vi "Main.vi"() -> ()   [LabVIEW 2019, in "Server.lvlib"]
doc: "This template is based off of the Queued Message Handler design pattern and the Queued Message Handler project template that ships with LabVIEW.\n\nThe main difference is that the queue is private to this module and communication between modules is performed via Broadcast and Request events.\n\nRequest events are wrapped in public API methods and are handled in the Event Handling Loop (EHL) of this VI. Any module can register for Broadcast events sent by this module. The EHL generates messages based on user interface actions.\n\nThe Message Handling Loop (MHL) processes messages generated by the EHL, or by other messages. The messages are string values, so new messages can be added easily to the Message Cases case structure in the MHL. Each message cluster can also provide an optional value for Message Data, which is a variant that can be converted to whatever message-specific data is required.\n_____\nBased on Delacor QMH Project Template 4.2.1.64."
uses:
  Server.lvlib
  <vilib>/Delacor/Delacor QMH/Libraries/Module Admin_class/Delacor_lib_QMH_Module Admin.lvclass
  Module Data--cluster.ctl
  <vilib>/Delacor/Delacor QMH/Libraries/Message Queue_class/Delacor_lib_QMH_Message Queue.lvclass/Delacor_lib_QMH_Message Queue.ctl
  Stop Argument--cluster.ctl
  <vilib>/Delacor/Delacor QMH/Libraries/Module Admin_class/Delacor_lib_QMH_Module Admin.lvclass/Delacor_lib_QMH_Module Admin.ctl
  <vilib>/Utility/miscctls.llb/LVPointTypeDef.ctl
  <vilib>/Delacor/Delacor QMH/Libraries/Message Queue_class/Delacor_lib_QMH_Enqueue Message (Single).vi
  <vilib>/Delacor/Delacor QMH/Libraries/Module Admin_class/Delacor_lib_QMH_Get External Launch.vi
  <vilib>/Utility/error.llb/Error Cluster From Error Code.vi
  <vilib>/ErrorRing/Error Ring.xnode
  <vilib>/Delacor/Delacor QMH/Libraries/Message Queue_class/Delacor_lib_QMH_Message Queue.lvclass
  Chat Window/Chat Window.lvlib
panel:
  in  "Chat Window Selection":i32(ring) items=["All"=-1]
  in  "Send Global Chat":bool
  in  "New Chat Window":bool
  in  "Send Message":string
  in  "Simulate MHL Error":bool
  in  "Simulate EHL Error":bool
  out "error out":errorcluster
  in  "Module Admin":refnum<class "Delacor_lib_QMH_Module Admin.lvclass">
  out "Status":string
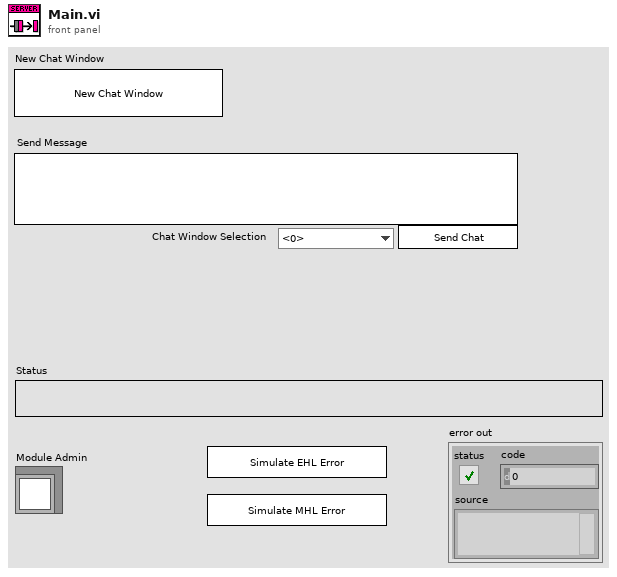
[diagram p1: front panel]
types:
  T1 = typedef "Chat Window.lvlib/Broadcast Events--cluster.ctl" = cluster{"Module Did Init":refnum<user-event>, "Status Updated":refnum<user-event>, "Error Reported":refnum<user-event>, "Module Did Stop":refnum<user-event>, "Update Module Execution Status":refnum<user-event>}
  T2 = typedef "Server.lvlib/Request Events--cluster.ctl" = cluster{"Stop Module":refnum<user-event>, "Show Panel":refnum<user-event>, "Hide Panel":refnum<user-event>, "Get Module Execution Status":refnum<user-event>, "Show Diagram":refnum<user-event>}
  T3 = typedef "Server.lvlib/Module Data--cluster.ctl" = cluster{"Status":string}
  T4 = enum32{"invalid lock state", "Not Locked", "Locked (No Password)", "Password-protected"}
  T5 = typedef "Server.lvlib/Stop Argument--cluster.ctl" = cluster{"Origin":string, "Exit via Stop Module Req?":bool, "Wait for Module to stop?":bool}
  T6 = typedef "LVPointTypeDef.ctl" = cluster{"Horizontal":i16, "Vertical":i16}
  T7 = enum32{"Invalid", "Standard", "Closed", "Hidden", "Minimized", "Maximized"}
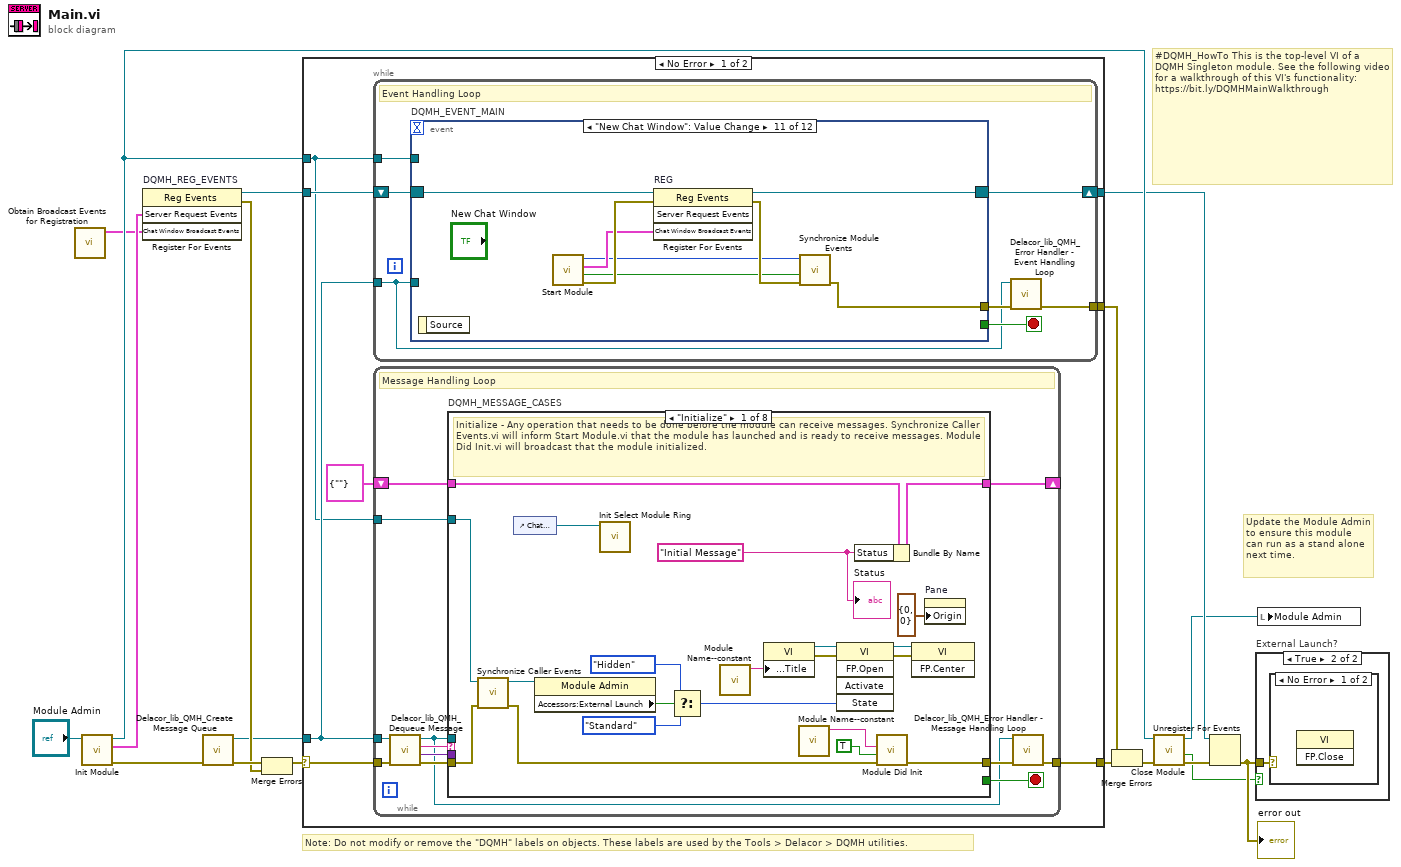
[diagram p0: block diagram]
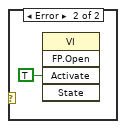
[diagram p3: hidden frame]
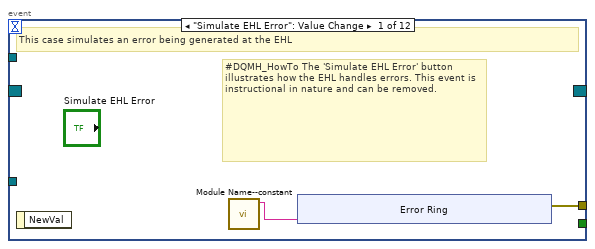
[diagram p4: hidden frame]
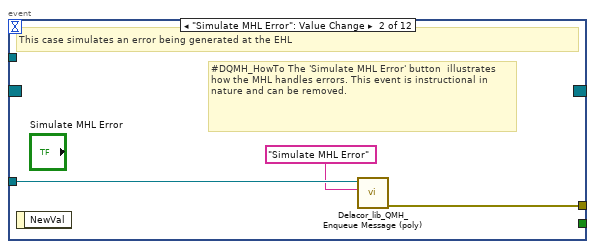
[diagram p5: hidden frame]
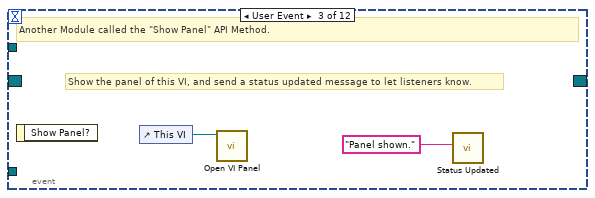
[diagram p6: hidden frame]
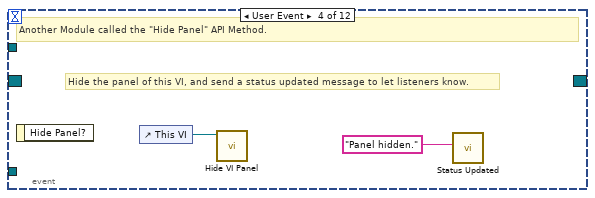
[diagram p7: hidden frame]
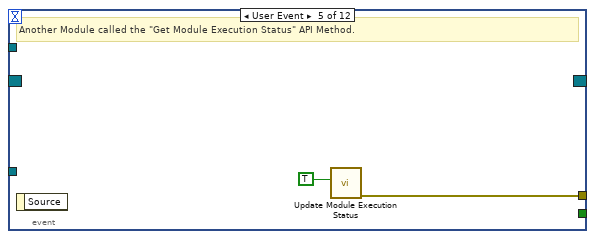
[diagram p8: hidden frame]
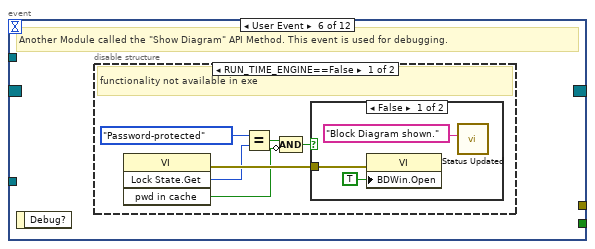
[diagram p9: hidden frame]
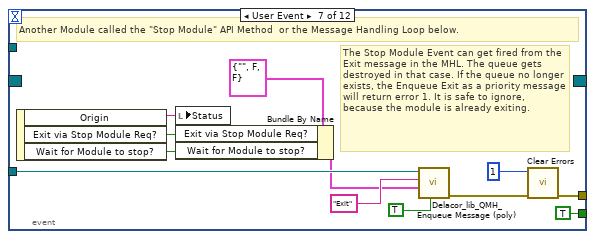
[diagram p12: hidden frame]
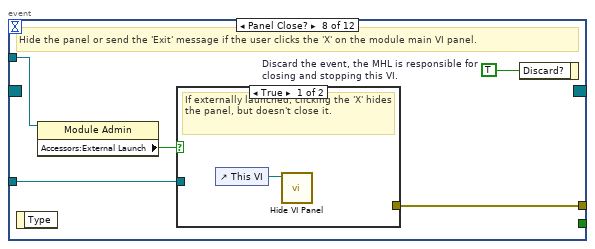
[diagram p13: hidden frame]
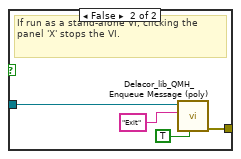
[diagram p14: hidden frame]
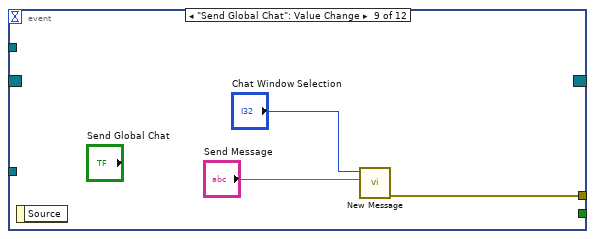
[diagram p15: hidden frame]
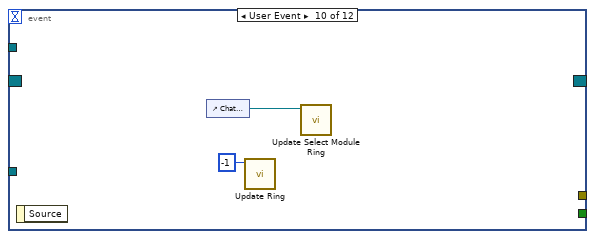
[diagram p16: hidden frame]
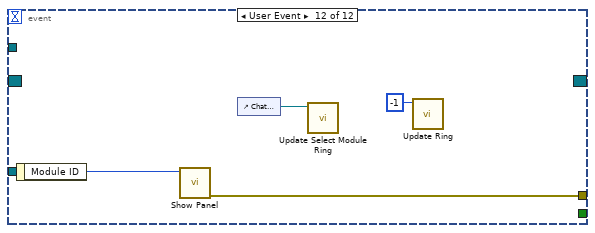
[diagram p17: hidden frame]
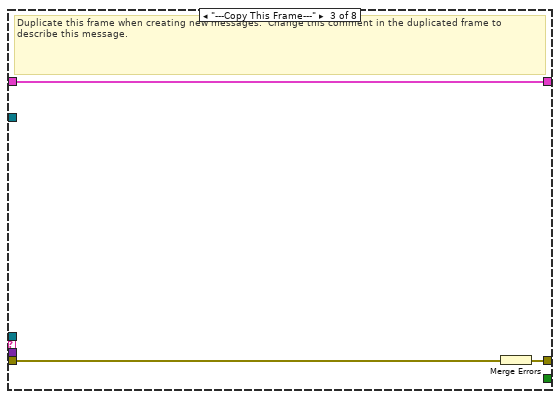
[diagram p19: hidden frame]
diagram:
  # "#DQMH_HowTo This is the top-level VI of a DQMH Singleton module. See the following video for a walkthrough of this VI's functionality: https://bit.ly/DQMHMainWalkthrough"
  # "Note: Do not modify or remove the \"DQMH\" labels on objects. These labels are used by the Tools > Delacor > DQMH utilities."
  # "Update the Module Admin to ensure this module can run as a stand alone next time."
  n1 = call "Obtain Broadcast Events for Registration.vi"() -> ("Chat Window Broadcast Events"=w1:T1)  [unwired: 10 in, 1 out]
  n2 = call "Init Module.vi"("Singleton Module Admin in"="Module Admin") -> ("error out"=w17:errorcluster, "Server Request Events"=w6:T2, "Singleton Module Admin out"=w9:refnum<class "Delacor_lib_QMH_Module Admin.lvclass">)  [unwired: 8 in]
  n3 = register-events "DQMH_REG_EVENTS"(w6, w1) -> (reference out=w7:refnum<event-registration>, error out=w10:errorcluster)  [unwired: 2 in]
  n4 = call <vilib>:"Delacor_lib_QMH_Create Message Queue.vi"("error in (no error)"=w17) -> ("error out"=w12:errorcluster, "Message Queue"=w5:refnum<class "Delacor_lib_QMH_Message Queue.lvclass">)  [unwired: 9 in]
  n5 = Merge Errors(w12, w10) -> (w11:errorcluster)
  n6 = case shown="No Error" w11 {
    selector: w11 -> [w24 w205]
    tunnel: [w26 w205] -> w18
    tunnel: [w23 w202] -> w8
    tunnel: w7 -> [w21 w202]
    tunnel: w5 -> [w20 _]
    tunnel: [w25 _] -> w15
    tunnel: w9 -> [w19 w198]
    frame No Error {
      n7 = while {
        tunnel: w20 -> [w27]
        shift-right: [w30] -> w23
        shift-left: w21 -> [w31]
        tunnel: [w32] -> w25
        tunnel: w19 -> [w28]
        stop <- w29 stop-if-true
        # "Event Handling Loop"
        n8 = event "DQMH_EVENT_MAIN" shown="[10] \"New Chat Window\": Value Change" {
          selector: w31 -> [_ _ _ _ _ _ _ _ _ _ w95 _]
          dyn-events: [_ _ _ _ _ _ _ _ _ _ w94 _] -> w30
          timeout: _ -> [_ _ _ _ _ _ _ _ _ _ _ _]
          tunnel: [_ _ _ _ _ _ TRUE ("Discard?") _ _ _ _ _] -> w29
          tunnel: w27 -> [_ w44 _ _ _ _ w68 w75 _ _ _ _]
          tunnel: [w35 w45 _ _ w51 _ w71 w77 w84 _ w88 w98] -> w33
          tunnel: w28 -> [_ _ _ _ _ _ _ w74 _ _ _ _]
          event "Simulate EHL Error": Value Change {
            # "#DQMH_HowTo The 'Simulate EHL Error' button  illustrates how the EHL handles errors. This event is instructional in nature and can be removed."
            # "This case simulates an error being generated at the EHL"
            n9 = event-data() -> ()  [unwired: 1 in, 1 out]
            n10 = call "Module Name--constant.vi"() -> ("Module Name"=w34:string)  [unwired: 11 in]
            n11 = xnode "Error Ring"("parameter 0"=w34) -> ("error out"=w35:errorcluster)
          }
          event "Simulate MHL Error": Value Change {
            # "#DQMH_HowTo The 'Simulate MHL Error' button  illustrates how the MHL handles errors. This event is instructional in nature and can be removed."
            # "This case simulates an error being generated at the EHL"
            n12 = event-data() -> ()  [unwired: 1 in, 1 out]
            n13 = call-poly <vilib>:"Delacor_lib_QMH_Enqueue Message (poly).vi"("Message"="Simulate MHL Error", "Message Queue in"=w44) -> ("error out"=w45:errorcluster)  [unwired: 8 in, 1 out]
          }
          event User Event {
            # "Show the panel of this VI, and send a status updated message to let listeners know."
            # "Another Module called the \"Show Panel\" API Method."
            n14 = event-data() -> ()  [unwired: 1 in, 1 out]
            n15 = control-ref of="This VI"() -> (w47:refnum<vi>)
            n16 = call "Open VI Panel.vi"("VI"=w47) -> ()  [unwired: 10 in, 1 out]
            n17 = call "Status Updated.vi"("Status"="Panel shown." ("format string")) -> ()  [unwired: 10 in, 1 out]
          }
          event User Event {
            # "Hide the panel of this VI, and send a status updated message to let listeners know."
            # "Another Module called the \"Hide Panel\" API Method."
            n18 = event-data() -> ()  [unwired: 1 in, 1 out]
            n19 = control-ref of="This VI"() -> (w49:refnum<vi>)
            n20 = call "Hide VI Panel.vi"("VI"=w49) -> ()  [unwired: 10 in, 1 out]
            n21 = call "Status Updated.vi"("Status"="Panel hidden." ("format string")) -> ()  [unwired: 10 in, 1 out]
          }
          event User Event {
            # "Another Module called the \"Get Module Execution Status\" API Method."
            n22 = event-data() -> ()  [unwired: 1 in, 1 out]
            n23 = call "Update Module Execution Status.vi"("Running?"=TRUE) -> ("error out"=w51:errorcluster)  [unwired: 10 in]
          }
          event User Event {
            # "Another Module called the \"Show Diagram\" API Method. This event is used for debugging."
            n24 = event-data() -> ()  [unwired: 1 in, 1 out]
            n25 = disable-structure shown="RUN_TIME_ENGINE==False" {
              frame condition #0 (active) {
                # "functionality not available in exe"
                n26 = invoke class="VI" method="Lock State.Get"() -> (error out=w57:errorcluster, "Get Lock State"=w56:T4, "pwd in cache"=w53:bool)  [unwired: 4 in, 1 out]
                n27 = Equal?(x=T4."Password-protected", y=w56) -> (x = y?=w54:bool)
                n28 = Compound Arithmetic op=AND(w54, invert w53) -> (w52:bool)
                n29 = case shown="False" w52 {
                  tunnel: w57 -> [w60 _]
                  frame False {
                    n30 = property class="VI"(error in=w60, "BDWin.Open"=TRUE ("Block Diagram Window:Open")) -> ()  [unwired: 1 in, 2 out]
                    n31 = call "Status Updated.vi"("Status"="Block Diagram shown." ("format string")) -> ()  [unwired: 10 in, 1 out]
                  }
                  frame True {
                    # "Password-protected VI, and the password is not in the cache. Do not show the diagram."
                  }
                }
              }
              frame condition #1 {
              }
            }
          }
          event User Event {
            # "The Stop Module Event can get fired from the Exit message in the MHL. The queue gets destroyed in that case. If the queue no longer exists, the Enqueue Exit as a priority message will return error 1. It is safe to ignore, because the module is already exiting."
            # "Another Module called the \"Stop Module\" API Method  or the Message Handling Loop below."
            n32 = event-data() -> ("Origin"=w67:string, "Exit via Stop Module Req?"=w63:bool, "Wait for Module to stop?"=w62:bool)  [unwired: 1 in]
            n33 = local write "Status"(w67) -> ()
            n34 = Bundle By Name(cluster=T5 {"Origin"="", "Exit via Stop Module Req?"=FALSE, "Wait for Module to stop?"=FALSE} ("Stop Argument"), "Exit via Stop Module Req?"=w63, "Wait for Module to stop?"=w62) -> (w61:T5)
            n35 = call-poly <vilib>:"Delacor_lib_QMH_Enqueue Message (poly).vi"("Priority Message? (F)"=TRUE, "Message Data"=w61, "Message"="Exit", "Message Queue in"=w68) -> ("error out"=w72:errorcluster)  [unwired: 6 in, 1 out]
            n36 = call <vilib>:"Clear Errors.vi"("error in (no error)"=w72, "specific error code to clear (0: all)"=1) -> ("error out"=w71:errorcluster)  [unwired: 4 in, 1 out]
          }
          event Panel Close? {
            w76 = TRUE  # Discard the event, the MHL is responsible for closing and stopping this VI.
            # "Hide the panel or send the 'Exit' message if the user clicks the 'X' on the module main VI panel."
            n37 = event-data() -> ()  [unwired: 1 in, 1 out]
            n38 = property class="Module Admin"(reference=w74) -> ("Accessors:External Launch"=w73:bool)  [unwired: 1 in, 2 out]
            n39 = case shown="True" w73 {
              tunnel: w75 -> [_ w81]
              tunnel: [_ w82] -> w77
              frame True {
                # "If externally launched, clicking the 'X' hides the panel, but doesn't close it."
                n40 = control-ref of="This VI"() -> (w78:refnum<vi>)
                n41 = call "Hide VI Panel.vi"("VI"=w78) -> ()  [unwired: 10 in, 1 out]
              }
              frame False {
                # "If run as a stand-alone VI, clicking the panel 'X' stops the VI."
                n42 = call-poly <vilib>:"Delacor_lib_QMH_Enqueue Message (poly).vi"("Priority Message? (F)"=TRUE, "Message"="Exit", "Message Queue in"=w81) -> ("error out"=w82:errorcluster)  [unwired: 7 in, 1 out]
              }
            }
            n43 = event-data("Discard?"=w76) -> ()  [unwired: 1 in, 1 out]
          }
          event "Send Global Chat": Value Change {
            n44 = event-data() -> ()  [unwired: 1 in, 1 out]
            n45 = call "New Message.vi"("Chat Message"="Send Message", "Module ID"="Chat Window Selection") -> ("error out"=w84:errorcluster)  [unwired: 9 in]
          }
          event User Event {
            n46 = event-data() -> ()  [unwired: 1 in, 1 out]
            n47 = control-ref of="Chat Window Selection"() -> (w87:refnum<vi>)
            n48 = call "Update Ring.vi"("Module ID"=-1) -> ()  [unwired: 10 in, 1 out]
            n49 = call "Update Select Module Ring.vi"("Select Module Ring Ref"=w87) -> ()  [unwired: 8 in, 3 out]
          }
          event "New Chat Window": Value Change {
            n50 = event-data() -> ()  [unwired: 1 in, 1 out]
            n51 = call "Start Module.vi"() -> ("error out"=w93:errorcluster, "Wait for Event Sync?"=w89:bool, "Chat Window Broadcast Events"=w91:T1, "Module ID"=w90:i32)  [unwired: 8 in]
            n52 = register-events "REG"(reference=w95, error in=w93, w91) -> (reference out=w94:refnum<event-registration>, error out=w92:errorcluster)  [unwired: 1 in]
            n53 = call "Synchronize Module Events.vi"("error in (no error)"=w92, "Wait for Event Sync?"=w89, "Module ID"=w90) -> ("error out"=w88:errorcluster)  [unwired: 7 in, 1 out]
          }
          event User Event {
            n54 = event-data() -> ("Module ID"=w99:i32)  [unwired: 1 in]
            n55 = call "Show Panel.vi"("Module ID"=w99) -> ("error out"=w98:errorcluster)  [unwired: 10 in]
            n56 = control-ref of="Chat Window Selection"() -> (w97:refnum<vi>)
            n57 = call "Update Select Module Ring.vi"("Select Module Ring Ref"=w97) -> ()  [unwired: 8 in, 3 out]
            n58 = call "Update Ring.vi"("Module ID"=-1) -> ()  [unwired: 10 in, 1 out]
          }
        }
        n59 = call-dynamic "Delacor_lib_QMH_Error Handler - Event Handling Loop.vi"("error in (no error)"=w33, "Message Queue in"=w27) -> ("dup error in"=w32:errorcluster)  [unwired: 8 in, 1 out]
      }
      n60 = while {
        tunnel: w20 -> [w102]
        shift-right: [w106] -> _
        shift-left: T3 {"Status"=""} ("Data Cluster") -> [w107]
        tunnel: w24 -> [w110]
        tunnel: [w108] -> w26
        tunnel: w19 -> [w100]
        stop <- w105 stop-if-true
        # "Message Handling Loop"
        n61 = call-dynamic "Delacor_lib_QMH_Dequeue Message.vi"("error in (no error)"=w110, "Message Queue in"=w102) -> ("error out"=w109:errorcluster, "Message Data"=w103:variant, "Message"=w104:string, "Message Queue out"=w101:refnum<class "Delacor_lib_QMH_Message Queue.lvclass">)  [unwired: 6 in]
        n62 = case "DQMH_MESSAGE_CASES" shown="\"Initialize\"" w104 {
          selector: w104 -> [_ _ _ _ _ _ _ w185]
          tunnel: w101 -> [_ _ _ _ _ w154 w177 _]
          tunnel: w109 -> [w130 w134 w137 w139 w144 w161 w183 w187]
          tunnel: [w128 w134 w136 w139 w143 w157 w180 w188] -> w111
          tunnel: w107 -> [w119 w133 w135 w138 w141 w156 w176 w186]
          tunnel: [w118 w133 w135 w138 w141 w156 w176 w186] -> w106
          tunnel: [_ _ _ _ _ _ w175 _] -> w105
          tunnel: w103 -> [_ _ _ _ _ w155 w174 _]
          tunnel: w100 -> [w120 _ _ _ _ w153 w169 _]
          frame "Initialize" {
            w113 = "Initial Message" ("Initial Message")
            # "Initialize - Any operation that needs to be done before the module can receive messages. Synchronize Caller Events.vi will inform Start Module.vi that the module has launched and is ready to receive messages. Module Did Init.vi will broadcast that the module initialized."
            n63 = call "Synchronize Caller Events.vi"("error in (no error)"=w130, "Singleton Module Admin in"=w120) -> ("error out"=w129:errorcluster, "Singleton Module Admin out"=w115:refnum<class "Delacor_lib_QMH_Module Admin.lvclass">)  [unwired: 8 in]
            n64 = control-ref of="Chat Window Selection"() -> (w112:refnum<vi>)
            n65 = property class="Module Admin"(reference=w115) -> ("Accessors:External Launch"=w124:bool)  [unwired: 1 in, 2 out]
            n66 = call "Init Select Module Ring.vi"("Select Module Ring Ref"=w112) -> ()  [unwired: 8 in, 3 out]
            n67 = Select(t=T7."Hidden" ("State"), s=w124, f=T7."Standard" ("State")) -> (s? t:f=w121:T7)
            n68 = call "Module Name--constant.vi"() -> ("Module Name"=w127:string)  [unwired: 11 in]
            n69 = property class="VI"("Front Panel.Title"=w127) -> (reference out=w126:refnum<vi>, error out=w132:errorcluster)  [unwired: 2 in]
            n70 = call "Module Name--constant.vi"() -> ("Module Name"=w116:string)  [unwired: 11 in]
            n71 = invoke class="VI" method="FP.Open"(reference=w126, error in=w132, "State"=w121) -> (reference out=w125:refnum<vi>, error out=w131:errorcluster)  [unwired: 2 in, 3 out]
            n72 = Bundle By Name(cluster=w119, "Status"=w113) -> (w118:T3)
            n73 = call "Module Did Init.vi"("error in (no error)"=w129, "Initialized?"=TRUE, "Origin"=w116) -> ("error out"=w128:errorcluster)  [unwired: 8 in]
            n74 = invoke class="VI" method="FP.Center"(reference=w125, error in=w131) -> ()  [unwired: 1 in, 3 out]
            n75 = property on="Pane" class="Pane"("Origin"=T6 {"Horizontal"=0, "Vertical"=0}) -> ()  [unwired: 2 in, 2 out]
            "Status" <- w113
          }
          frame "--- Module Specific ---" {
            # "Separator -- The following cases handle messages specific to this Module."
          }
          frame "---Copy This Frame---" {
            # "Duplicate this frame when creating new messages.  Change this comment in the duplicated frame to describe this message."
            n76 = Merge Errors(w137) -> (w136:errorcluster)
          }
          frame "--- Exit and Error Handling---" {
            # "Separator - The following cases handle errors and exit messages."
          }
          frame "Simulate MHL Error" {
            # "#DQMH_HowTo The 'Simulate MHL Error' button  illustrates how the MHL handles errors. This event is instructional in nature and can be removed."
            # "Simulate an error occurring at the MHL"
            n77 = call "Module Name--constant.vi"() -> ("Module Name"=w140:string)  [unwired: 11 in]
            n78 = xnode "Error Ring"("parameter 0"=w140) -> ("error out"=w142:errorcluster)
            n79 = Merge Errors(w144, w142) -> (w143:errorcluster)
          }
          frame "Error" {
            # "#CodeRecommended - If you ever change the name of this \"Error\" message, you'll need to update the name in the Check Loop Error.vi as well."
            # "#CodeRecommended - If the module is running in standalone mode (External Launch = FALSE), this code will pop up an error dialog and call the 'Exit' message if an error occurs. Add more fine-grained error handling here."
            # "Error - Check the error message data and respond accordingly. This message is sent by the \"Error Handler\" VIs at the end of each loop in this application."
            n80 = property class="Module Admin"(reference=w153) -> ("Accessors:External Launch"=w152:bool)  [unwired: 1 in, 2 out]
            n81 = Variant To Data(error in=w161, type=errorcluster {"status"=FALSE, "code"=0, "source"=""} ("error constant"), Variant=w155) -> (data=w162:errorcluster, error out=w159:errorcluster)
            n82 = call "Error Reported.vi"("Error"=w162) -> ()  [unwired: 10 in, 1 out]
            n83 = case shown="False" w152 {
              tunnel: [w167 _] -> w158
              tunnel: w154 -> [w165 _]
              tunnel: w162 -> [w166 _]
              frame False {
                # "If the module is running standalone, then pop up an error dialog and call the \"Exit\" message."
                n84 = call <vilib>:"Simple Error Handler.vi"("error in (no error)"=w166) -> ()  [unwired: 4 in, 5 out]
                n85 = call-poly <vilib>:"Delacor_lib_QMH_Enqueue Message (poly).vi"("Priority Message? (F)"=TRUE, "Message"="Exit", "Message Queue in"=w165) -> ("error out"=w167:errorcluster)  [unwired: 7 in, 1 out]
              }
              frame True {
                # "If the module was launched externally, calling the Error Reported broadcast VI is the only action performed by the \"Error\" message. The module's caller can then process the error appropriately."
              }
            }
            n86 = Merge Errors(w159, w158) -> (w157:errorcluster)
            n87 = local write "error out"(w157) -> ()
          }
          frame "Exit" {
            w173 = 91  # 91: not all Exit messages will have an argument
            w175 = TRUE  # Stop the VI
            # "Release the message queue reference"
            # "#CodeNeeded - Add any required cleanup code here"
            # "Exit - Exit the application."
            n88 = Variant To Data(error in=w183, type=T5 {"Origin"="", "Exit via Stop Module Req?"=FALSE, "Wait for Module to stop?"=FALSE} ("Stop Argument"), Variant=w174) -> (data=w171:T5, error out=w179:errorcluster)
            n89 = call <vilib>:"Clear Errors.vi"("error in (no error)"=w179, "specific error code to clear (0: all)"=w173) -> ("error out"=w182:errorcluster)  [unwired: 4 in, 1 out]
            n90 = control-ref of="This VI"() -> (w170:refnum<vi>)
            n91 = call-dynamic "Delacor_lib_QMH_Release Message Queue.vi"("error in (no error)"=w182, "Message Queue"=w177) -> ("error out"=w181:errorcluster)  [unwired: 9 in]
            n92 = call "Handle Exit.vi"("Stop Argument"=w171, "Admin in"=w169, "VI reference"=w170) -> ("error out"=w178:errorcluster)  [unwired: 7 in, 1 out]
            n93 = Merge Errors(w181, w178) -> (w180:errorcluster)
            n94 = call "Stop Module.vi"("Module ID"=-1) -> ()  [unwired: 10 in, 1 out]
          }
          frame Default {
            # "'Default' case only runs if there is a message that isn't defined in any of the other cases.  Output a programming error."
            n95 = call "Module Name--constant.vi"() -> ("Module Name"=w184:string)  [unwired: 11 in]
            n96 = xnode "Error Ring"("parameter 0"=w185, "parameter 1"=w184) -> ("error out"=w189:errorcluster)
            n97 = Merge Errors(w187, w189) -> (w188:errorcluster)
          }
        }
        n98 = call-dynamic "Delacor_lib_QMH_Error Handler - Message Handling Loop.vi"("error in (no error)"=w111, "Message Queue in"=w101) -> ("dup error in"=w108:errorcluster)  [unwired: 8 in, 1 out]
      }
    }
    frame Error {
      # "Synchronize Caller Events.vi will inform Start Module.vi that the module has launched and will let the code calling Start Module.vi register for broadcasts and would permit the caller receive the broadcast that an error occurred at launch time."
      n99 = call "Synchronize Caller Events.vi"("Singleton Module Admin in"=w198) -> ("error out"=w203:errorcluster)  [unwired: 9 in, 1 out]
      n100 = call "Module Name--constant.vi"() -> ("Module Name"=w201:string)  [unwired: 11 in]
      n101 = Format Into String(format string="An error occurred during initialization. %s is no longer running.", w201) -> (resulting string=w199:string)  [unwired: 2 in, 1 out]
      n102 = Merge Errors(w205, w203) -> (w204:errorcluster)
      n103 = call "Error Reported.vi"("Additional Information"=w199, "Error"=w204) -> ()  [unwired: 9 in, 1 out]
    }
  }
  n104 = Merge Errors(w15, w18) -> (w14:errorcluster)
  n105 = call "Close Module.vi"("error in (no error)"=w14, "Module Admin in"=w9) -> ("error out"=w16:errorcluster, "External Launch"=w2:bool, "Module Admin out"=w3:refnum<class "Delacor_lib_QMH_Module Admin.lvclass">)  [unwired: 7 in]
  n106 = Unregister For Events(event registration refnum=w8, error in=w16) -> (error out=w13:errorcluster)
  "error out" <- w13
  n107 = case "External Launch?" shown="True" w2 {
    tunnel: w13 -> [_ w206]
    frame False {
    }
    frame True {
      n108 = case shown="No Error" w206 {
        frame No Error {
          n109 = invoke class="VI" method="FP.Close"() -> ()  [unwired: 3 in, 3 out]
        }
        frame Error {
          n110 = invoke class="VI" method="FP.Open"("Activate"=TRUE ("Activate?")) -> ()  [unwired: 4 in, 5 out]
        }
      }
    }
  }
  n111 = local write "Module Admin"(w3) -> ()
